vi "PH_uOPA_DelayController.handle Oscilloscope Signals.vi"(0 "VI in":refnum<vi>, 5 "error in":errorcluster) -> (14 "VI out":refnum<vi>, 19 "error out":errorcluster)   [LabVIEW 2014, in "PH_uOPA_DelayController.lvlib"]
uses:
  PH_uOPA_DelayController.lvlib
  PH_uOPA_DelayController.Control Status.ctl
  PH_Devices/PH_TKTDS-30xx/PH_TKTDS-30xx.lvlib
  PH_Basics/PH_Common/PH_Common.lvlib
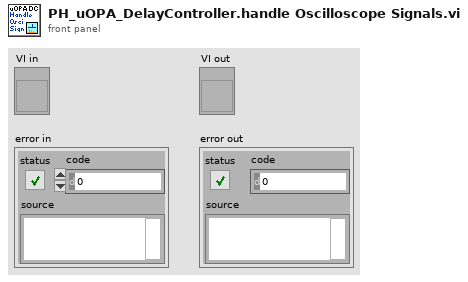
[diagram p1: front panel]
types:
  T1 = typedef "PH_uOPA_DelayController.lvlib/PH_uOPA_DelayController.i attribute.ctl" = cluster{"GUI Refs":cluster{"Current Pump Peak":refnum<vi>, "Current uOPA Peak":refnum<vi>, "Pump Peak":refnum<vi>, "uOPA Peak":refnum<vi>, "uOPA Target":refnum<vi>, "uOPA Limits [%]":refnum<vi>, "sample length":refnum<vi>, "Pump Target":refnum<vi>, "Pump Limit":refnum<vi>, "Pump running":refnum<vi>, "Feedback Control":refnum<vi>, "Control Status":refnum<vi>, "uOPA Mean":refnum<vi>, "Current uOPA Mean":refnum<vi>}, "uOPA Target":dbl, "uOPA Limits [%]":T2, "Sample Length":i32, "Initialize Mean":bool, "Pump Target":dbl, "Pump Limit [%]":dbl, "Feedback Control":bool, "Control Status":T3, "last Mean":dbl, "last direction":T4, "Axis Settings":T5, "Width while feedback":dbl}
  T2 = typedef "PH_uOPA_DelayController.lvlib/PH_uOPA_DelayController.Limit.ctl" = cluster{"low":dbl, "activate":dbl, "fine":dbl}
  T3 = typedef "PH_uOPA_DelayController.lvlib/PH_uOPA_DelayController.Control Status.ctl" = enum32{"off", "Pump off", "calculating", "too low", "activated", "fine"}
  T4 = typedef "PH_Stepmotor_BaseClass.lvlib/PH_Stepmotor_BaseClass.Axis Direction.ctl" = enum16{"forward", "backward"}
  T5 = typedef "PH_Stepmotor_BaseClass.lvlib/PH_Stepmotor_BaseClass.Axis Settings.ctl" = cluster{"Sign change":bool, "Width":dbl, "Calibration":dbl, "Unit":string, "Motor Type":T6, "Unit Width":string, "Unit CF":string}
  T6 = typedef "PH_Stepmotor_BaseClass.lvlib/PH_Stepmotor_BaseClass.Motor Type.ctl" = enum16{"Unspecific", "OWIS 49.120.2633", "OWIS 49.060.1033", "OWIS 43.040.2558", "Diamond Motion 2200 series", "OWIS 49.120.266B.MV6", "Calorimeter", "Linear Stage 1", "MICOS VT-80", "MICOS VT-80 S", "Standa Rotstage nt0.95A", "PUF RA 320.200", "PUF RA 800.200", "PUF RA 800.400", "PUF RA 400.50", "1324.nn.800.50", "1324.n9c.800.50", "1324.nn.320.200", "1324.nn.400.200", "1324.nn.800.200", "1324.nn.400.50", "1324.8c9c.800.50", "1324.8c9c.400.200"}
  T7 = typedef "PH_TKTDS-30xx.lvlib/PH_TKTDS-30xx.i attribute.ctl" = cluster{"Default VISA Resource":string, "VISA Resource Name":refnum<visa-resource-name>, "Revision":cluster{"Instrument Driver":string, "Instrument Firmware":string}, "Selftest":cluster{"Result":u32, "Message":string}, "Channels":T8[], "Trigger Configuration":T10, "Acquisition Configuration":T11, "Fetched Waveforms":T12[], "GUI Refs":T13, "State":T14, "Error Message":string, "Allow Prdc Loop?":bool}
  T8 = typedef "PH_TKTDS-30xx.lvlib/PH_TKTDS-30xx.Channel Config.ctl" = cluster{"Channel Name":string, "Input Impedance":string, "Max Input Frequency":string, "Vertical Coupling":i32, "Channel Enabled":bool, "Probe Attenuation":dbl, "Vertical Range":dbl, "Vertical Offset":dbl, "Waveform Limits":T9}
  T9 = typedef "PH_TKTDS-30xx.lvlib/PH_TKTDS-30xx.Waveform Limits.ctl" = cluster{"Start":i32, "End":i32}
  T10 = typedef "PH_TKTDS-30xx.lvlib/PH_TKTDS-30xx.Trigger Config.ctl" = cluster{"Source":string, "Slope":i32, "Level [V]":dbl}
  T11 = typedef "PH_TKTDS-30xx.lvlib/PH_TKTDS-30xx.Acquisition Config.ctl" = cluster{"Time base":dbl, "Record Length":u16, "Start Time":dbl, "Type":i32, "Continuous":bool}
  T12 = typedef "PH_TKTDS-30xx.lvlib/PH_TKTDS-30xx.fetched Waveform.ctl" = cluster{"Source":string, "Actual Points":u32, "Initial X":dbl, "X Increment":dbl, "Waveform Array":dbl[]}
  T13 = typedef "PH_TKTDS-30xx.lvlib/PH_TKTDS-30xx.GUI Refs.ctl" = cluster{"Trigger":refnum<vi>, "Acquisition":refnum<vi>, "State":refnum<vi>, "Delete":refnum<vi>, "Channel to be positioned":refnum<vi>, "Postion":refnum<vi>, "Display Intensity":refnum<vi>, "VISA Resource":refnum<vi>, "Channels":refnum<vi>[], "Graphs":refnum<vi>[]}
  T14 = typedef "PH_StatusHandler.lvlib/PH_StatusHandler.Status.ctl" = i16
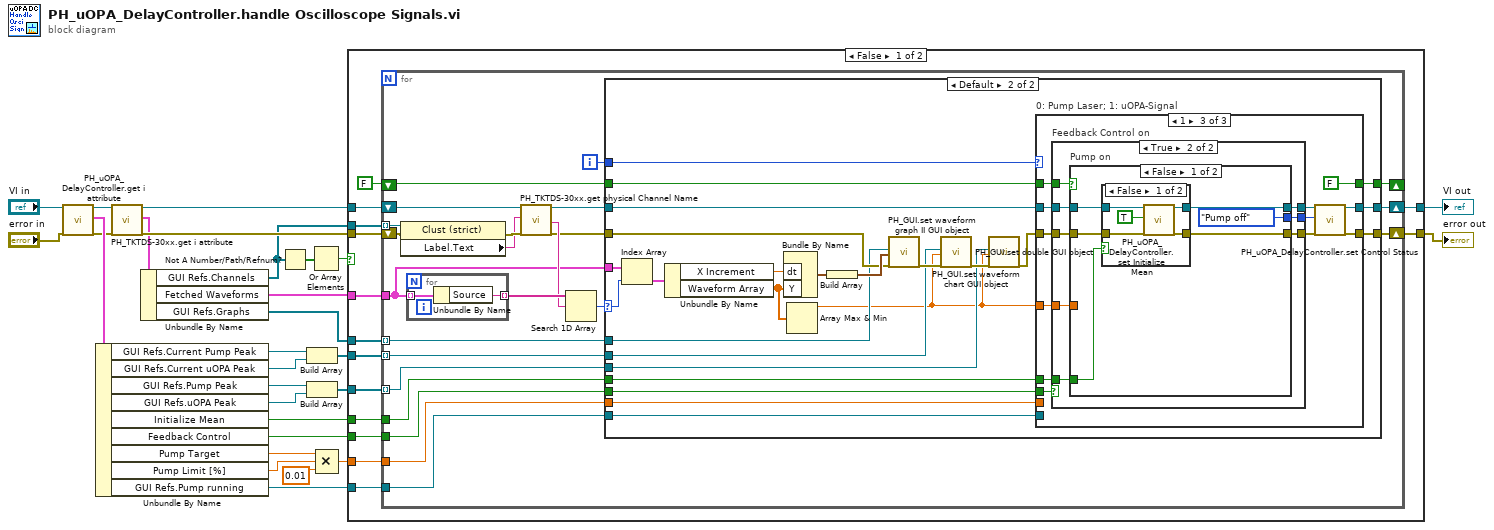
[diagram p0: block diagram]
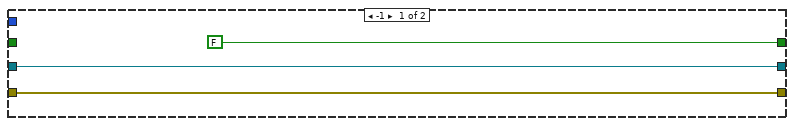
[diagram p2: hidden frame]
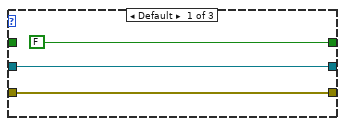
[diagram p3: hidden frame]
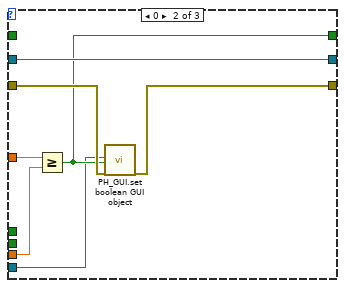
[diagram p4: hidden frame]
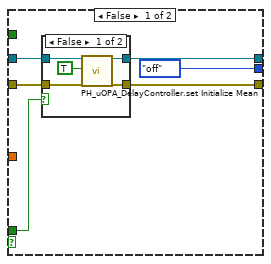
[diagram p5: hidden frame]
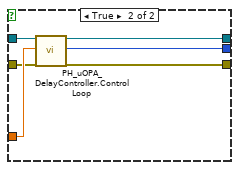
[diagram p8: hidden frame]
diagram:
  n1 = call "PH_uOPA_DelayController.get i attribute.vi"("i ref in"="VI in", "error in (no error)"="error in") -> ("i ref out"=w13:refnum<vi>, "i attribute"=w14:T1, "error out"=w12:errorcluster)  [unwired: 15 in]
  n2 = Unbundle By Name(w14) -> ("GUI Refs.Current Pump Peak"=w15:refnum<vi>, "GUI Refs.Current uOPA Peak"=w16:refnum<vi>, "GUI Refs.Pump Peak"=w17:refnum<vi>, "GUI Refs.uOPA Peak"=w18:refnum<vi>, "Initialize Mean"=w2:bool, "Feedback Control"=w28:bool, "Pump Target"=w24:dbl, "Pump Limit [%]"=w25:dbl, "GUI Refs.Pump running"=w1:refnum<vi>)
  n3 = call "PH_TKTDS-30xx.get i attribute.vi"("i ref in"=w13, "error in (no error)"=w12) -> ("i ref out"=w10:refnum<vi>, "i attribute"=w4:T7, "error out"=w11:errorcluster)  [unwired: 15 in]
  n4 = Unbundle By Name(w4) -> ("GUI Refs.Channels"=w9:refnum<vi>[], "Fetched Waveforms"=w3:T12[], "GUI Refs.Graphs"=w23:refnum<vi>[])
  n5 = Not A Number/Path/Refnum?(number/path/refnum=w9) -> (NaN/Path/Refnum?=w7:bool[])
  n6 = Build Array(w15, w16) -> (w19:refnum<vi>[])
  n7 = Build Array(w17, w18) -> (w20:refnum<vi>[])
  n8 = Or Array Elements(Boolean array=w7) -> (logical OR=w8:bool)
  n9 = Compound Arithmetic op=MULTIPLY(w24, w25, 0.01 ("value")) -> (w26:dbl)
  n10 = case shown="False" w8 {
    tunnel: w3 -> [w42 _]
    tunnel: w10 -> [w39 w159]
    tunnel: w11 -> [w41 w158]
    tunnel: [w38 w159] -> w5
    tunnel: [w37 w158] -> w6
    tunnel: w9 -> [w40 _]
    tunnel: w23 -> [w36 _]
    tunnel: w19 -> [w35 _]
    tunnel: w20 -> [w34 _]
    tunnel: w2 -> [w33 _]
    tunnel: w26 -> [w32 _]
    tunnel: w28 -> [w30 _]
    tunnel: w1 -> [w29 _]
    frame False {
      n11 = for {
        tunnel: w42 -> [w57]
        shift-right: [w55] -> w37
        shift-left: w41 -> [w63]
        tunnel: w40 -> [w62] mode=indexing
        shift-right: [w49] -> w38
        shift-left: w39 -> [w59]
        tunnel: w36 -> [w54] mode=indexing
        tunnel: w35 -> [w53] mode=indexing
        tunnel: w34 -> [w52] mode=indexing
        tunnel: w33 -> [w51]
        tunnel: w32 -> [w47]
        shift-right: [w46] -> _
        shift-left: FALSE -> [w45]
        tunnel: w30 -> [w44]
        tunnel: w29 -> [w43]
        i -> [w48]
        n12 = property class="Clust (strict)"(reference=w62, error in=w63) -> (error out=w61:errorcluster, "Label.Text"=w60:string)  [unwired: 1 out]
        n13 = for {
          tunnel: w57 -> [w157] mode=indexing
          tunnel: [w156] -> w64 mode=indexing
          n14 = Unbundle By Name(w157) -> ("Source"=w156:string)
        }
        n15 = call "PH_TKTDS-30xx.get physical Channel Name.vi"("i ref in"=w59, "GUI Element Name"=w60, "error in"=w61) -> ("i ref out"=w50:refnum<vi>, "Physical Channel Name"=w58:string, "error out"=w56:errorcluster)  [unwired: 13 in, 1 out]
        n16 = Search 1D Array(1D array=w64, element=w58) -> (index of element=w65:i32)  [unwired: 1 in]
        n17 = case shown="Default" w65 {
          selector: w65 -> [_ w91]
          tunnel: w57 -> [_ w93]
          tunnel: w56 -> [w68 w87]
          tunnel: [w68 w79] -> w55
          tunnel: w54 -> [_ w80]
          tunnel: w53 -> [_ w84]
          tunnel: w52 -> [_ w81]
          tunnel: w51 -> [_ w76]
          tunnel: w50 -> [w67 w78]
          tunnel: [w67 w77] -> w49
          tunnel: w48 -> [_ w75]
          tunnel: w47 -> [_ w69]
          tunnel: [FALSE w74] -> w46
          tunnel: w45 -> [_ w73]
          tunnel: w43 -> [_ w72]
          tunnel: w44 -> [_ w71]
          frame -1 {
          }
          frame Default {
            n18 = Index Array(array=w93, index=w91) -> (element=w92:T12)
            n19 = Unbundle By Name(w92) -> ("X Increment"=w90:dbl, "Waveform Array"=w85:dbl[])
            n20 = Bundle By Name("dt"=w90, "Y"=w85) -> (w89:waveform(dbl))  [unwired: 1 in]
            n21 = Array Max & Min(array=w85) -> (max value=w70:dbl)  [unwired: 3 out]
            n22 = Build Array(w89) -> (w88:waveform(dbl)[])
            n23 = call "PH_GUI.set waveform graph II GUI object.vi"("WaveformGraph in"=w80, "Array"=w88, "error in (no error)"=w87) -> ("error out"=w86:errorcluster)  [unwired: 16 in]
            n24 = call "PH_GUI.set double GUI object.vi"("GUI object Ref"=w84, "value"=w70, "error in (no error)"=w86) -> ("error out"=w83:errorcluster)  [unwired: 16 in]
            n25 = call "PH_GUI.set waveform chart GUI object.vi"("WaveformChart in"=w81, "Double"=w70, "error in (no error)"=w83) -> ("error out"=w82:errorcluster)  [unwired: 16 in]
            n26 = case "0: Pump Laser; 1: uOPA-Signal" shown="1" w75 {
              tunnel: w82 -> [w95 w100 w115]
              tunnel: w70 -> [_ w103 w114]
              tunnel: [w95 w99 w108] -> w79
              tunnel: w78 -> [w96 w101 w112]
              tunnel: [w96 w101 w106] -> w77
              tunnel: w76 -> [_ _ w111]
              tunnel: w69 -> [_ w102 _]
              tunnel: [FALSE w98 FALSE] -> w74
              tunnel: w73 -> [_ _ w109]
              tunnel: w72 -> [_ w97 _]
              tunnel: w71 -> [_ _ w104]
              frame Default {
              }
              frame 0 {
                n27 = Greater Or Equal?(x=w103, y=w102) -> (x >= y?=w98:bool)
                n28 = call "PH_GUI.set boolean GUI object.vi"("Boolean Knob GUI Ref"=w97, "Value"=w98, "error in (no error)"=w100) -> ("error out"=w99:errorcluster)  [unwired: 16 in]
              }
              frame 1 {
                n29 = case "Feedback Control on" shown="True" w104 {
                  tunnel: w115 -> [w119 w136]
                  tunnel: w114 -> [_ w135]
                  tunnel: [w117 w134] -> w113
                  tunnel: w112 -> [w121 w133]
                  tunnel: w111 -> [w118 w132]
                  tunnel: w109 -> [_ w131]
                  tunnel: [w120 w130] -> w107
                  tunnel: [PH_uOPA_DelayController.Control_Status."off" ("Control Status") w129] -> w105
                  frame False {
                    n30 = case shown="False" w118 {
                      tunnel: w119 -> [w126 w127]
                      tunnel: [w125 w127] -> w117
                      tunnel: w121 -> [w124 w128]
                      tunnel: [w123 w128] -> w120
                      frame False {
                        n31 = call "PH_uOPA_DelayController.set Initialize Mean.vi"("VI in"=w124, "Initialize Mean? (True)"=TRUE, "error in (no error)"=w126) -> ("VI out"=w123:refnum<vi>, "error out"=w125:errorcluster)  [unwired: 15 in]
                      }
                      frame True {
                      }
                    }
                  }
                  frame True {
                    n32 = case "Pump on" shown="False" w131 {
                      tunnel: w136 -> [w140 w151]
                      tunnel: w135 -> [_ w154]
                      tunnel: [w139 w152] -> w134
                      tunnel: w133 -> [w142 w150]
                      tunnel: [w141 w155] -> w130
                      tunnel: w132 -> [w138 _]
                      tunnel: [PH_uOPA_DelayController.Control_Status."Pump off" ("Control Status") w153] -> w129
                      frame False {
                        n33 = case shown="False" w138 {
                          tunnel: w140 -> [w147 w148]
                          tunnel: [w146 w148] -> w139
                          tunnel: w142 -> [w145 w149]
                          tunnel: [w144 w149] -> w141
                          frame False {
                            n34 = call "PH_uOPA_DelayController.set Initialize Mean.vi"("VI in"=w145, "Initialize Mean? (True)"=TRUE, "error in (no error)"=w147) -> ("VI out"=w144:refnum<vi>, "error out"=w146:errorcluster)  [unwired: 15 in]
                          }
                          frame True {
                          }
                        }
                      }
                      frame True {
                        n35 = call "PH_uOPA_DelayController.Control Loop.vi"("VI in"=w150, "uOPA Peak"=w154, "error in (no error)"=w151) -> ("VI out"=w155:refnum<vi>, "Control Status"=w153:T3, "error out"=w152:errorcluster)  [unwired: 14 in]
                      }
                    }
                  }
                }
                n36 = call "PH_uOPA_DelayController.set Control Status.vi"("VI in"=w107, "Control Status"=w105, "error in (no error)"=w113) -> ("VI out"=w106:refnum<vi>, "error out"=w108:errorcluster)  [unwired: 15 in]
              }
            }
          }
        }
      }
    }
    frame True {
    }
  }
  "error out" <- w6
  "VI out" <- w5
